vi "Diff_MNU.vi"() -> ()   [LabVIEW 2017]
panel:
  in  "File 1":string
  in  "File 2":string
  in  "error out":errorcluster
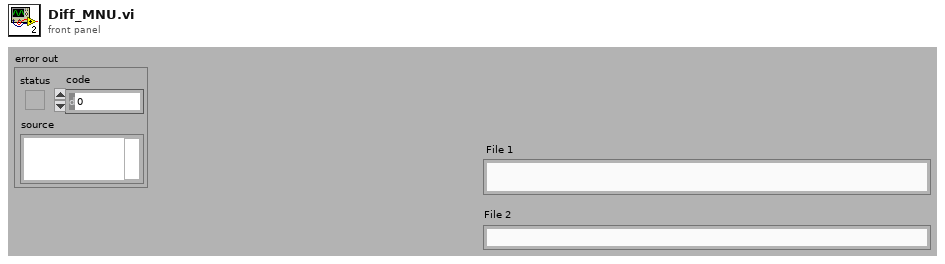
[diagram p1: front panel]
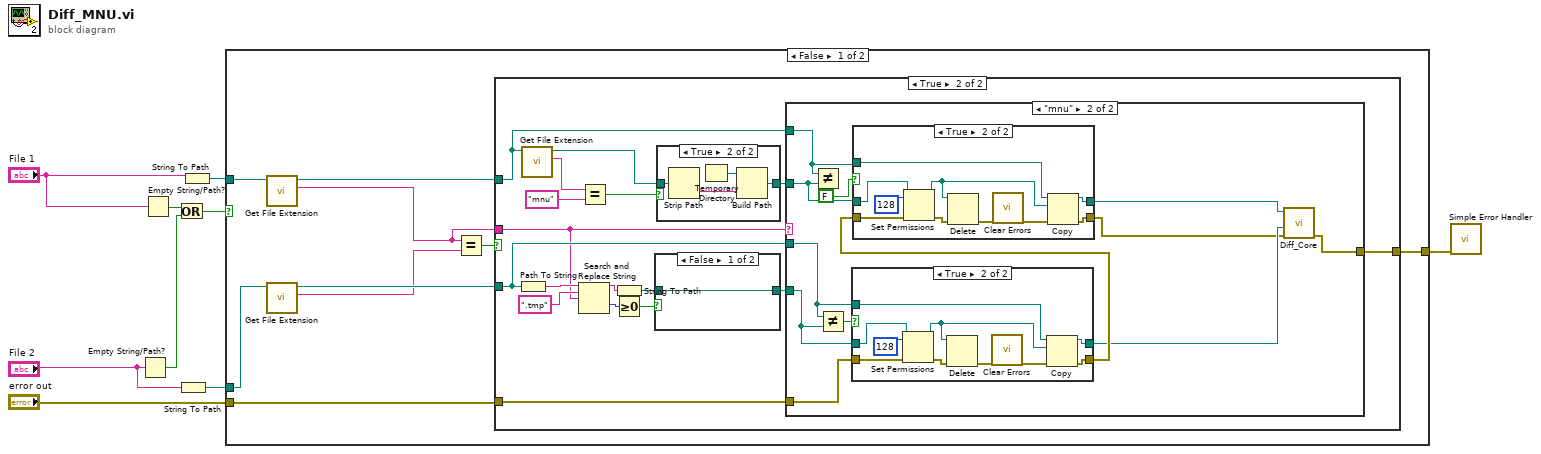
[diagram p0: block diagram]
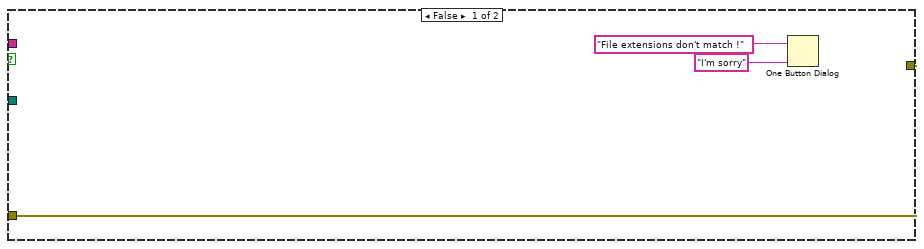
[diagram p2: hidden frame]
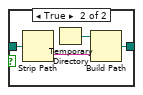
[diagram p3: hidden frame]
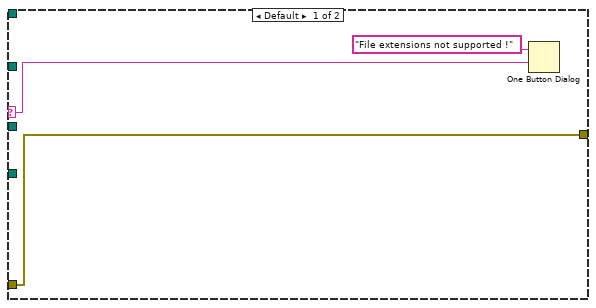
[diagram p5: hidden frame]
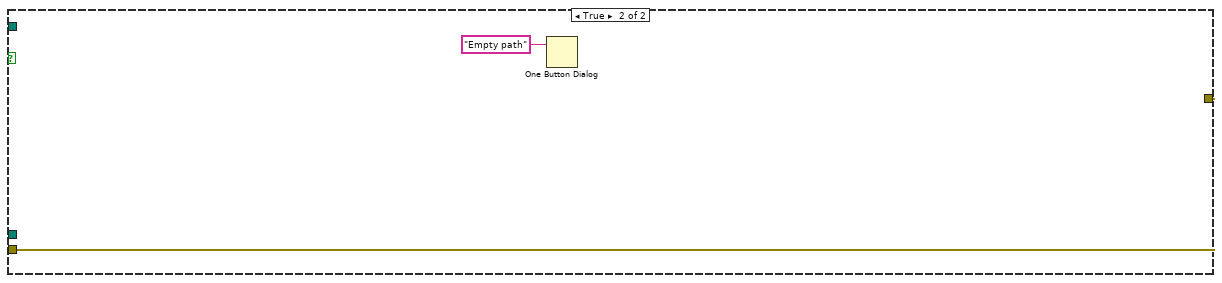
[diagram p8: hidden frame]
diagram:
  n1 = Empty String/Path?(string/path="File 2") -> (empty?=w5:bool)
  n2 = Empty String/Path?(string/path="File 1") -> (empty?=w6:bool)
  n3 = Or(x=w6, y=w5) -> (x .or. y?=w4:bool)
  n4 = String To Path(string="File 2") -> (path=w9:path)
  n5 = String To Path(string="File 1") -> (path=w8:path)
  n6 = case shown="False" w4 {
    tunnel: w9 -> [w16 _]
    tunnel: w8 -> [w13 _]
    tunnel: "error out" -> [w18 w89]
    tunnel: [w17 w89] -> w7
    frame False {
      n7 = call <vilib>:"Get File Extension.vi"("file"=w13) -> ("lowercase file extension"=w10:string, "dup file"=w12:path)  [unwired: 1 in, 8 out]
      n8 = call <vilib>:"Get File Extension.vi"("file"=w16) -> ("lowercase file extension"=w14:string, "dup file"=w15:path)  [unwired: 1 in, 8 out]
      n9 = Equal?(x=w10, y=w14) -> (x = y?=w11:bool)
      n10 = case shown="True" w11 {
        tunnel: w18 -> [w19 w38]
        tunnel: w12 -> [_ w27]
        tunnel: w15 -> [_ w34]
        tunnel: w10 -> [_ w22]
        tunnel: [w19 w28] -> w17
        frame False {
          n11 = One Button Dialog(message="File extensions don't match !", button name ("OK")="I'm sorry") -> ()  [unwired: 1 out]
        }
        frame True {
          n12 = Path To String(path=w34) -> (string=w37:string)
          n13 = call <vilib>:"Get File Extension.vi"("file"=w27) -> ("lowercase file extension"=w25:string, "dup file"=w26:path)  [unwired: 1 in, 8 out]
          n14 = Search and Replace String(input string=w37, search string=".tmp" ("y"), replace string=w22) -> (result string=w35:string, offset past replacement=w30:i32)  [unwired: 1 in, 6 out]
          n15 = Equal?(x=w25, y="mnu") -> (x = y?=w23:bool)
          n16 = String To Path(string=w35) -> (path=w32:path)
          n17 = Greater Or Equal To 0?(x=w30) -> (x >= 0?=w29:bool)
          n18 = case shown="False" w29 {
            tunnel: w32 -> [w39 w41]
            tunnel: [w39 w40] -> w31
            frame False {
            }
            frame True {
              n19 = Strip Path(path=w41) -> (name=w42:string)  [unwired: 1 out]
              n20 = Temporary Directory() -> (w43:path)
              n21 = Build Path(base path=w43, name or relative path=w42) -> (appended path=w40:path)
            }
          }
          n22 = case shown="True" w23 {
            tunnel: w26 -> [w44 w48]
            tunnel: [w44 w45] -> w33
            frame False {
            }
            frame True {
              n23 = Strip Path(path=w48) -> (name=w47:string)  [unwired: 1 out]
              n24 = Temporary Directory() -> (w46:path)
              n25 = Build Path(base path=w46, name or relative path=w47) -> (appended path=w45:path)
            }
          }
          n26 = case shown="\"mnu\"" w22 {
            selector: w22 -> [w49 _]
            tunnel: w38 -> [w50 w57]
            tunnel: w27 -> [_ w60]
            tunnel: w34 -> [_ w62]
            tunnel: w31 -> [_ w61]
            tunnel: w33 -> [_ w59]
            tunnel: [w50 w53] -> w28
            frame Default {
              n27 = One Button Dialog(message="File extensions not supported !", button name ("OK")=w49) -> ()  [unwired: 1 out]
            }
            frame "mnu" {
              n28 = Not Equal?(x=w60, y=w59) -> ()  [unwired: 1 out]
              n29 = Not Equal?(x=w62, y=w61) -> (x != y?=w63:bool)
              n30 = case shown="True" w63 {
                tunnel: w61 -> [_ w78]
                tunnel: w57 -> [w77 w82]
                tunnel: w62 -> [w76 w85]
                tunnel: [w77 w84] -> w58
                tunnel: [w76 w83] -> w55
                frame False {
                }
                frame True {
                  n31 = Set Permissions(7:i16 128 ("new permissions"), 8:w82, 11:w78) -> (0:w81:errorcluster, 3:w80:path)  [unwired: 2 out]
                  n32 = Delete(path (use dialog)=w80, error in=w81) -> (error out=w87:errorcluster)  [unwired: 5 out]
                  n33 = call <vilib>:"Clear Errors.vi"("error in (no error)"=w87) -> ("error out"=w86:errorcluster)  [unwired: 1 in, 5 out]
                  n34 = Copy(8:w86, 10:w80, 11:w85) -> (0:w84:errorcluster, 3:w83:path)  [unwired: 3 out]
                }
              }
              n35 = case shown="True" FALSE {
                tunnel: w59 -> [_ w66]
                tunnel: w58 -> [w65 w70]
                tunnel: w60 -> [w64 w73]
                tunnel: [w65 w72] -> w54
                tunnel: [w64 w71] -> w56
                frame False {
                }
                frame True {
                  n36 = Set Permissions(7:i16 128 ("new permissions"), 8:w70, 11:w66) -> (0:w69:errorcluster, 3:w68:path)  [unwired: 2 out]
                  n37 = Delete(path (use dialog)=w68, error in=w69) -> (error out=w75:errorcluster)  [unwired: 5 out]
                  n38 = call <vilib>:"Clear Errors.vi"("error in (no error)"=w75) -> ("error out"=w74:errorcluster)  [unwired: 1 in, 5 out]
                  n39 = Copy(8:w74, 10:w68, 11:w73) -> (0:w72:errorcluster, 3:w71:path)  [unwired: 3 out]
                }
              }
              n40 = call "Diff_Core.vi"("error in (no error)"=w54, "palette path 2"=w55, "palette path  1"=w56) -> ("error out"=w53:errorcluster)  [unwired: 8 out]
            }
          }
        }
      }
    }
    frame True {
      n41 = One Button Dialog(message="Empty path") -> ()  [unwired: 2 out]
    }
  }
  n42 = call <vilib>:"Simple Error Handler.vi"("error in (no error)"=w7) -> ()  [unwired: 1 in, 8 out]
